vi "sv_Non Causal Propagation Padding .vi"(7 "frequency to generate [Hz]":dbl format="%.2f", 10 "AI sampling frequency":dbl format="%.2f", 11 "indice computations in":T1) -> (3 "indice computations in":T1)   [LabVIEW 2017, in "SoundVib_SweptSine.lvlib"]
uses:
  <vilib>/addons/Sound and Vibration/svt_Swept Sine/SoundVib_SweptSine.lvlib
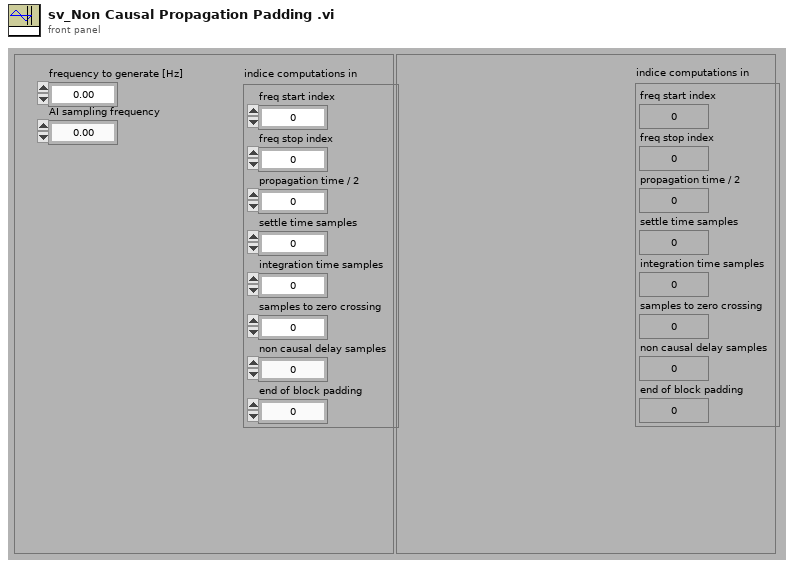
[diagram p1: front panel]
types:
  T1 = cluster{"freq start index":u32, "freq stop index":u32, "propagation time / 2":u32, "settle time samples":u32, "integration time samples":u32, "samples to zero crossing":u32, "non causal delay samples":u32, "end of block padding":u32}
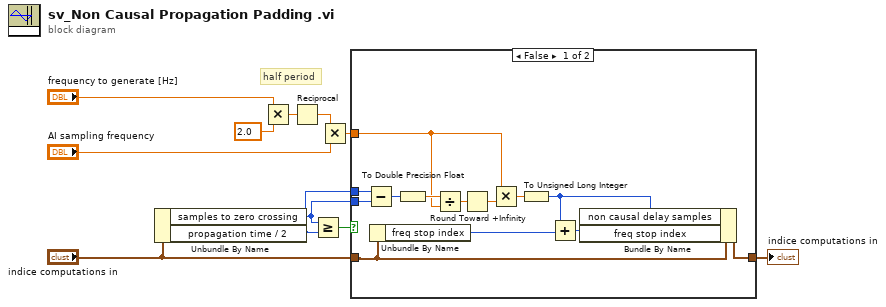
[diagram p0: block diagram]
diagram:
  # "half period"
  n1 = Unbundle By Name("indice computations in") -> ("samples to zero crossing"=w7:u32, "propagation time / 2"=w6:u32)
  n2 = Multiply(x="frequency to generate [Hz]", y=2.0) -> (x*y=w8:dbl)
  n3 = Reciprocal(x=w8) -> (1/x=w5:dbl)
  n4 = Greater Or Equal?(x=w7, y=w6) -> (x >= y?=w11:bool)
  n5 = Multiply(x=w5, y="AI sampling frequency") -> (x*y=w10:dbl)
  n6 = case shown="False" w11 {
    tunnel: w6 -> [w24 _]
    tunnel: w7 -> [w23 _]
    tunnel: w10 -> [w18 _]
    tunnel: "indice computations in" -> [w14 w25]
    tunnel: [w13 w25] -> w2
    frame False {
      n7 = Subtract(x=w24, y=w23) -> (x-y=w22:u32)
      n8 = Unbundle By Name(w14) -> ("freq stop index"=w16:u32)
      n9 = To Double Precision Float(number=w22) -> (double precision float=w21:dbl)
      n10 = Divide(x=w21, y=w18) -> (x/y=w20:dbl)
      n11 = Round Toward +Infinity(x=w20) -> (ceil(x): smallest int >= x=w17:dbl)
      n12 = Multiply(x=w18, y=w17) -> (x*y=w19:dbl)
      n13 = To Unsigned Long Integer(number=w19) -> (unsigned 32bit integer=w12:u32)
      n14 = Add(x=w12, y=w16) -> (x+y=w15:u32)
      n15 = Bundle By Name(cluster=w14, "non causal delay samples"=w12, "freq stop index"=w15) -> (w13:T1)
    }
    frame True {
    }
  }
  "indice computations in" <- w2
